vi "AlliGator Run FLI Dataset Python Function.vi"(8 "error in (no error)":errorcluster, 9 "Current Data":string, 10 "Python Function Info":T1={"Script Path"=path "", "Function Name"="", "Function Parent Menu"="", "Function Input Parameters"=[], "Function Outputs"=[], "Function Doc String"="", "Function Display Name"="", "Function Target Type"=enum."Window Menu", "Function Target Window"="", "Parent Menu Location"="", "Item Menu Tag"="", "Is preceded by Separator"=FALSE}, 11 "Data Value Reference in":refnum<data-value>) -> (0 "error out":errorcluster, 1 "Message":string, 2 "Function Output Destination":string, 3 "Data Value Reference out":refnum<data-value>)   [LabVIEW 2021, in "AlliGator Python Plugins.lvlib"]
doc: "Runs FLI Dataset python plugin function."
uses:
  AlliGator Python Plugins.lvlib
  AlliGator Internal Variables v2.ctl
  <vilib>/vision/Image Controls.llb/IMAQ Image.ctl
  AlliGator Gate Image Set.ctl
  AlliGator FLI Dataset Type.ctl
  AlliGator Data Series Type.ctl
  AlliGator Dataset Channel.ctl
  AlliGator Gate Arithmetic.ctl
  AlliGator Displayed Image.ctl
  Image/Named ROI Description.ctl
  AlliGator Decay Metadata v3.ctl
  AlliGator Decay Background Subtraction Info.ctl
  AlliGator Baseline Subtraction Method.ctl
  Graphs/XY Graph/XY Graph Plot Shift Parameters.ctl
  Graphs/XY Graph/XY Graph Plot Shift Method.ctl
  AlliGator Decay Extrapolation Parameters.ctl
  Phasor/Calibration Phasor (m, phi).ctl
  Phasor/Phasor Reference Series.ctl
  Phasor/Phasor Calibration Map v2.ctl
  Phasor/Phasor (g, s).ctl
  AlliGator Raw Phasor Plot Data v4.ctl
  Phasor/Phasor Standard Deviation Options.ctl
  AlliGator Phasor Multi-Harmonic Data.ctl
  Phasor/Phasor Harmonic Data.ctl
  AlliGator Decay Fit Options & Parameters v2.ctl
  Fits/IRF(X)PSED/Decay Fit Options v2.ctl
  Fits/Decay Convolution/Decay Model.ctl
  Fits/Residual Type.ctl
  Fits/IRF(X)PSED/Fit Weights Type.ctl
  Fits/Non-linear Fitting Method v2.ctl
  Fits/Fit Calculation Method.ctl
  Fits/Non-linear Fitting Algorithm.ctl
  AlliGator Decay Fit Parameter Constraints 2.ctl
  Fits/IRF(X)PSED/Decay Fit Parameters In List.ctl
  Fits/IRF(X)PSED/MLE Baseline Offset Type.ctl
  AlliGator Decay Preprocessing Parameters.ctl
  Fits/IRF(X)PSED/Decay Fit Parameters & Derived Quantities List.ctl
  AlliGator Python Function Information.ctl
  AlliGator Python Function Parameter Definition.ctl
  AlliGator Python Function Output Definition.ctl
  AlliGator Python Plugin Target Type.ctl
  AlliGator Variables List.ctl
  AlliGator Python Plugin FLI Dataset Data.ctl
  AlliGator Python Plugin Image Data.ctl
  AlliGator Python Plugin Plot Data.ctl
  AlliGator Python Plugin Parameter Map Data.ctl
  Image/Image Point.ctl
  <vilib>/Utility/error.llb/Error Cluster From Error Code.vi
  <vilib>/ErrorRing/Error Ring.xnode
  AlliGator Globals, Variables & Constants.lvlib
  Image/Image.lvlib
  Strings/Strings.lvlib
  Error/Error.lvlib
  Phasor/Phasor.lvlib
  AlliGator Decay Preprocessing.lvlib
  Graphs/XY Graph/XY Graph Add-Ons.lvlib
  AlliGator Phasor Graph.lvlib
  AlliGator Files.lvlib
  AlliGator Phasor Plot.lvlib
  AlliGator Source Image.lvlib
  Fits/Fits.lvlib
  AlliGator Decay Fit.lvlib
  AlliGator Decay Fit Parameter Map.lvlib
  AlliGator Internal Variables.lvlib
  AlliGator Settings.lvlib
  AlliGator Dual-Channel Datasets.lvlib
panel:
  out "session out":refnum<k35>
  out "Function Parameters String":string
  # "see the AlliGator License on the block diagram (Ctrl+E or Window:Show Block Diagram)"
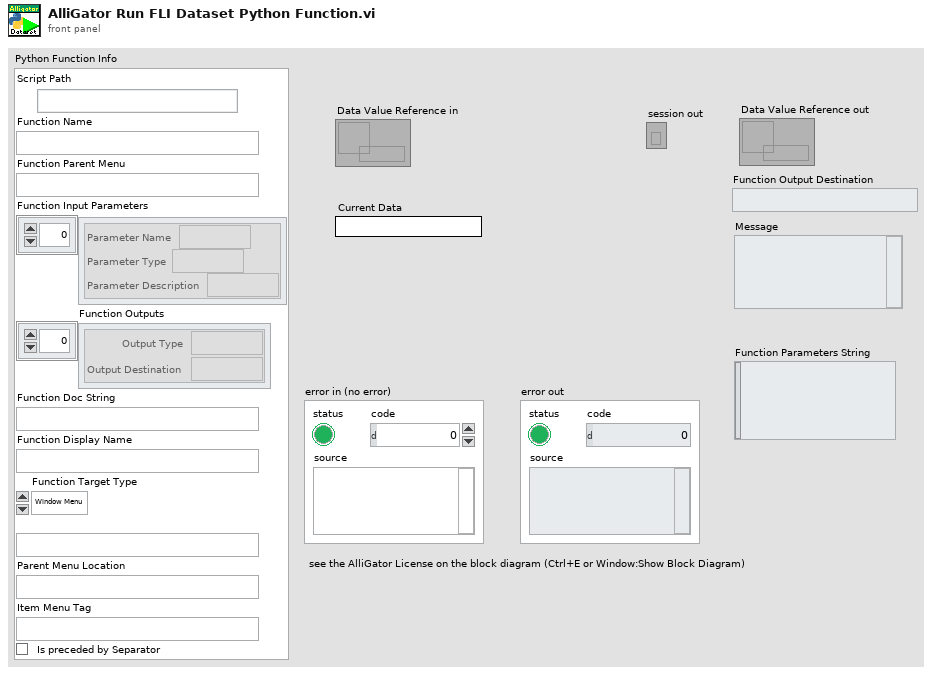
[diagram p1: front panel]
types:
  T1 = typedef "AlliGator Python Plugins.lvlib/AlliGator Python Function Information.ctl" = cluster{"Script Path":path, "Function Name":string, "Function Parent Menu":string, "Function Input Parameters":T2[], "Function Outputs":T3[], "Function Doc String":string, "Function Display Name":string, "Function Target Type":T4, "Function Target Window":string, "Parent Menu Location":string, "Item Menu Tag":string, "Is preceded by Separator":bool}
  T2 = typedef "AlliGator Python Plugins.lvlib/AlliGator Python Function Parameter Definition.ctl" = cluster{"Parameter Name":string, "Parameter Type":string, "Parameter Description":string}
  T3 = typedef "AlliGator Python Plugins.lvlib/AlliGator Python Function Output Definition.ctl" = cluster{"Output Type":string, "Output Destination":string}
  T4 = typedef "AlliGator Python Plugins.lvlib/AlliGator Python Plugin Target Type.ctl" = enum16{"Undefined", "Window Menu", "Object Menu"}
  T5 = typedef "AlliGator Python Plugins.lvlib/AlliGator Python Plugin FLI Dataset Data.ctl" = cluster{"FLI_Dataset_Name":string, "Gate_Duration":dbl, "Gate_Separation":dbl, "Gate_Number":u32, "X_Size":i32, "Y_Size":i32, "Image_Data_List":T6[], "Reference_Decay":T7, "Mask_Image":i32[][], "Parameter_Map":T8}
  T6 = typedef "AlliGator Python Plugins.lvlib/AlliGator Python Plugin Image Data.ctl" = cluster{"Image_Name":string, "Image":sgl[][]}
  T7 = typedef "AlliGator Python Plugins.lvlib/AlliGator Python Plugin Plot Data.ctl" = cluster{"Plot_Name":string, "X_Array":dbl[], "Y_Array":dbl[]}
  T8 = typedef "AlliGator Python Plugins.lvlib/AlliGator Python Plugin Parameter Map Data.ctl" = cluster{"Parameter_Names":string[], "Parameter_Flattened_Map":dbl[][], "Locations":T9[], "IRF_X":dbl[], "IRF_Y_Flattened_List":dbl[][]}
  T9 = typedef "Image.lvlib/Image Point.ctl" = cluster{"X":i32, "Y":i32}
  T10 = typedef "AlliGator Globals, Variables & Constants.lvlib/AlliGator Variables List.ctl" = enum16{"---- GUI ----", "Initialization Status", "State Indicators Refnum", "Original AlliGator Menu Items", "Current Action Loop State", "Script in progress", "Playback", "Loop Playback", "Search ROI Used", "Search ROI", "Decay Graph Max Legend Size", "Intensity Graph Max Legend Size", "Decay Statistics Graph Max Legend Size", "Phasor Graph Max Legend Size", "Phasor Ratio Graph Max Legend Size", "Lifetime Graph Max Legend Size", "---- Files ----", "Export Dataset Frames as Individual Files", "Show Batch Export Help Balloons", "Frames in Dataset", "ptu File Frame Start Indices", "Current Frame in Dataset", "Current Frame Timestamp", "------ Python Plugins ------", "Python Plugins Information", "Python Session", "Valid Python Session?", "---- Source Image ----", "Dataset Loaded", "Dataset Metadata", "Dataset Channel", "Dataset Data Description", "Background Dataset Metadata", "Background Dataset Channel", "Background Dataset Data Description", "Background File Subtraction", "Background File Path", "Background File Pile-up Correction", "Background File Pixel Well Capacity", "Background File Scaling Factor", "Source Image ROIs", "Current Source Image ROI", "Source Image ROI Event Refnum", "X_Source Image Display Range", "X_Source Image Palette Information", "Source Image Palette List", "Source Image Scale", "Current Dataset Load Settings", "Source Image:ROI Overlay Color", "---- Image Profile Window ----", "Image Profile:Overlay ROI in Source Image", "Image Profile Window Event Refnum", "Image Profile:IntensityType", "Image Profile:Intensity Average Type", "Image Profile:Intensity-weighted SDV", "Image Profile:Box Profile Type", "Image Profile Window Open", "Image Profile:Plotted Fit Parameter", "X_Type of Displayed Image", "X_Time Gate Slider", "Dataset Path", "Source Image Overlay to Erase", "Is Displayed Image Accumulated", "White Light Image Modified", "Mask Image Modified", "Macrotime Gate Separation", "------ Phasor Graph -------", "Phasor Graph:Show Line", "---- Phasor Plot ---", "Phasor Plot Parameters Changed", "FLI Dataset Modified since last Phasor Plot Calculation", "Phasor Harmonics Data", "Selected Phasor Harmonics", "Phasor Harmonic Manager Event Refnum", "Phasor Plot ROIs", "Current Phasor Plot ROI", "Phasor Plot ROI Event Refnum", "Phasor Plot Image Reference Points", "Phasor Plot Computed", "Phasor Plot Palette Information", "Phasor Plot Palette List", "Phasor Ratio Palette Information", "Phasor Ratio Palette List", "Phasor Image Scale", "Phasor Plot Image Overlay to Erase", "Phasor Plot Image Elements to Update", "Current Phasor Plot Calculation Parameters", "Current Phasor Calibration Options", "Reset Cumulated Phasor Plot", "Phasor Ratio Reference 1", "Phasor Ratio Lifetime Reference 1", "Phasor Ratio Reference 1 Frequency", "Phasor Ratio Reference 2", "Phasor Ratio Lifetime Reference 2", "Phasor Ratio Reference 2 Frequency", "---- Decay Analysis ----", "Number of Selected Decays to Fit", "LS Fit Results", "LAR Fit Results", "BS Fit Results", "Last Decay Max - Min", "Best Fit Parameters", "Best Fit Parameter Names", "Actual Size X", "Actual Size Y", "Binning X", "Binning Y", "Actual # Gates", "Dataset Number", "Gates to...", "Gates Skipped", "Gates to keep", "Gate Step", "Gate Separation", "Reversed Gates", "Pile-up Correction", "Pixel Well Capacity", "Background Subtracted", "Background Subtraction Method", "Background Definition Range", "Background File (deprecated)", "Number of Dataset Accumulated", "Array of Accumulated Dataset Paths", "Do Averaged Datasets", "Destination File Path", "Process Plot Target", "Use 1/D as Phasor Frequency", "---- Decay Fit Parameter Map -----", "Decay Fit Parameter Map Palette Information", "Decay Fit Parameter Map Palette List", "Local Decay Graph Window Event Refnum", "------- Local Decay Window ---------", "Use normalized IRF for convolution", "----- Miscellaneous ----", "Skippable Dialog Windows Status"}
  T11 = typedef "AlliGator Internal Variables.lvlib/AlliGator Internal Variables v2.ctl" = cluster{"Displayed Image":T12, "White Light Image":T12, "Mask Image":T12, "ROI Mask Image":T12, "Current Dataset Images 1":T13, "Background Dataset Images 1":T13, "Current Dataset Images 2":T13, "Background Dataset Images 2":T13, "Current Dataset Arithmetic Images":T13, "Accumulated Dataset Images 1":T13, "Accumulated Dataset Images 2":T13, "Accumulated Dataset Arithmetic Images":T13, "Phasor Plot Image":T12, "Decay Fit Parameter Map Image":T12, "Single Data Point Path":path, "White Light Image Path":path, "Mask Image Path":path, "Time-Series Folder":path, "[Time-Series Paths]":path[], "Current Dataset":i32, "Single Dataset Type":T14, "Current Folder":string, "AlliGator Data Series Type":T15, "# Datasets":i32, "Dual-Channel Dataset":bool, "Selected Channel Name":string, "Dataset Channel":T16, "Channel Arithmetic":T17, "Dual-Channel Background Dataset":bool, "Background Channel":T16, "Dual-Channel Accumulated Dataset":bool, "Start Time":dbl, "[Time-Series Timestamps]":dbl[], "[Intensity Corrections]":dbl[], "Time Series Script":bool, "Type of Displayed Image":T18, "Gate Image Slide":u16, "# Gates":i32, "ROIs":T19[], "ROI Decay":cluster{"t Array":dbl[], "I Array":dbl[]}, "Valid Decay":bool, "Decay  Metadata":T21, "Reference Decay Plot Name":string, "Reference Decay":cluster{"t Array":dbl[], "I Array":dbl[]}, "Decay Shift Plot":cluster{"Time Stamps":dbl[], "Decay Shifts":dbl[]}, "[Decays Max Values]":sgl[], "[Decays Min Values]":sgl[], "Calibration Phasor":T27, "Calibration Phasor Series":T28, "Phasor Calibration Map":T29, "Calibration Map MD5 Digest":string, "Last Raw Phasor":T30, "Last Calibrated Phasor":T30, "Last Calibrated Phasor SDV":T30, "Phasor Graph:Phasor Plot":cluster{"g Array":dbl[], "s Array":dbl[]}, "Phasor Graph:Phasor SDV Plot":cluster{"g Array":dbl[], "s Array":dbl[]}, "[Phasor Graph:Raw Phasor Plots]":T31[], "Phasor Plot locked to Ref 1":i32, "[Phasor Plot(s) locked to Ref 1]":i32[], "[Phasor Plot(s) locked to Ref 2]":i32[], "[Pixel Phasors]":T30[], "[[Sum Image]]":dbl[][], "[[CSG Phasors]]":csg[][], "[[Valid Pixel?]]":bool[][], "I/m/phi Dataset":cluster{"I/m/phi Dataset?":bool, "Base Frequency":dbl[unit], "Harmonic Orders":u8[]}, "Multi Phasor Plot Data":T33, "Decay Fit Options & Parameters":T35, "Fit Options: Decay Preprocessing Parameters":T46, "Fit Options: Reference Decay":cluster{"t Array":dbl[], "I Array":dbl[]}, "Is Full Image Parameters Map":bool, "Is Single-Pixels Parameters Map":bool, "NLSF Parameters Map X Resolution":i32, "NLSF Parameters Map Y Resolution":i32, "[Single Decay Fit Parameters]":dbl[], "Fit Model":T37, "[[Multiple Decays Fit Parameters]]":dbl[][], "[[Multiple Decays Fit Parameter SDVs]]":dbl[][], "[[IRFs]]":dbl[][], "IRF Array Time Axis":dbl[], "Decay Array Time Axis":dbl[], "[Decay Fit Parameter Names]":T47[], "[[Phasor Ratios]]":dbl[][], "[[Average Lifetimes]]":dbl[][], "Amplitude Weighted Average Lifetime":bool, "[Decay Sum]":dbl[], "[[User-defined Quantities]]":dbl[][], "User-defined Quantity":string}
  T12 = typedef "IMAQ Image.ctl" = refnum<image>
  T13 = typedef "AlliGator Files.lvlib/AlliGator Gate Image Set.ctl" = cluster{"SGL Image Max":T12, "SGL Image Sum":T12, "SGL Gate Images":T12[], "SGL Image Min":T12}
  T14 = typedef "AlliGator Files.lvlib/AlliGator FLI Dataset Type.ctl" = enum16{"HDF5 FLI Dataset", "Gate Image Folder", ".sdt FLI Dataset (Becker & Hickl)", ".ptu FLI Dataset (PicoQuant)", "SS1 FLI Dataset", "SS2 FLI Dataset", "I/m/phi Dataset", ".bin FLI Dataset (PicoQuant Binned)", ".bin FLI Dataset (Piccolo Binned)"}
  T15 = typedef "AlliGator Files.lvlib/AlliGator Data Series Type.ctl" = enum16{"Not a Supported Series", "Gate Images Folder Series", "SwissSPAD 2 Dataset Series", "B&H FLI Dataset Series", "PicoQuant PTU FLI Dataset Series", "PicoQuant BIN FLI Dataset Series", "Piccolo hist BIN FLI Dataset Series", "HDF5 FLI Dataset Series"}
  T16 = typedef "AlliGator Dual-Channel Datasets.lvlib/AlliGator Dataset Channel.ctl" = enum16{"G2", "INT"}
  T17 = typedef "AlliGator Settings.lvlib/AlliGator Gate Arithmetic.ctl" = enum16{"None", "INT-G2", "G2/INT*<INT>", "(1 - G2/INT)*<INT>"}
  T18 = typedef "AlliGator Source Image.lvlib/AlliGator Displayed Image.ctl" = enum16{"Single Gate", "Sum of All Gates", "Max of All Gates", "Min of All Gates", "-", "White Ligth Image", "Mask Image"}
  T19 = typedef "Image.lvlib/Named ROI Description.ctl" = cluster{"ROI Descriptor":T20, "ROI Name":string, "Overlay Color":u32}
  T20 = typedef "ROI Descriptor" = cluster{"Global Rectangle":i32[], "Contours":cluster{"ID":enum32{"External", "Internal"}, "Type":u32, "Coordinates":i32[]}[]}
  T21 = typedef "AlliGator Phasor Graph.lvlib/AlliGator Decay Metadata v3.ctl" = cluster{"ROI Descriptor":T20, "ROI Center":cluster{"X":i32, "Y":i32}, "Decay Background Subtraction Info":T22, "Decay Reverted":bool, "Decay Smoothened":bool, "Decay Straightened":bool, "Fitted Tau (Decay Straightening)":dbl, "Decay Shift Parameters":T24, "Decay Shifted":bool, "Decay Extrapolated":bool, "Decay Extrapolation Parameters":T26, "Decay Normalized":bool, "Fold Decay":bool, "# Folds":u32}
  T22 = typedef "AlliGator Decay Analysis.lvlib/AlliGator Decay Preprocessing.lvlib/AlliGator Decay Background Subtraction Info.ctl" = cluster{"Laser Period":dbl[unit], "Gate Duration":dbl[unit], "Baseline Subtraction Method":T23, "Background Definition Range":cluster{"Min Gate":dbl[unit], "Max Gate":dbl[unit]}, "Total Intensity w/o Bkgd Subtraction":dbl, "Bkgd-subtracted Intensity (exp)":dbl, "# Data Points":i32, "Background/Gate":dbl, "Fitted Lifetime":dbl[unit], "Bkgd-subtracted Intensity (theo)":dbl}
  T23 = typedef "AlliGator Decay Analysis.lvlib/AlliGator Decay Preprocessing.lvlib/AlliGator Baseline Subtraction Method.ctl" = enum16{"Mean", "Min", "Square Gated Single-Exponential", "File", "Constant"}
  T24 = typedef "XY Graph Add-Ons.lvlib/XY Graph Plot Shift Parameters.ctl" = cluster{"Type":T25, "Shift":dbl[unit], "Threshold":dbl, "Rotate":bool}
  T25 = typedef "XY Graph Add-Ons.lvlib/XY Graph Plot Shift Method.ctl" = enum16{"Default", "CFD", "Threshold", "Cross-Correlation"}
  T26 = typedef "AlliGator Decay Analysis.lvlib/AlliGator Decay Preprocessing.lvlib/AlliGator Decay Extrapolation Parameters.ctl" = cluster{"Additional Points":u32, "Head Fraction":dbl, "Fitted Tau":dbl, "Use Periodicity":bool, "Use Cursors":bool, "Tail Fraction":dbl}
  T27 = typedef "Phasor.lvlib/Calibration Phasor (m, phi).ctl" = cluster{"m":dbl, "phi":dbl, "Phasor Frequency":dbl[unit], "Reference Lifetime":dbl[unit]}
  T28 = typedef "Phasor.lvlib/Phasor Reference Series.ctl" = cluster{"m Array":dbl[], "phi Array":dbl[], "Phasor Frequency":dbl[unit], "Calibration Lifetime":dbl[unit]}
  T29 = typedef "AlliGator Phasor Calibration.lvlib/AlliGator Phasor Calibration Map v2.ctl" = cluster{"Phasor Frequency":dbl[unit], "Calibration Lifetime":dbl[unit], "ROI Centers":cluster{"X":i32, "Y":i32}[], "ROI Descriptors":T20[], "Map Resolution X":i32, "Map Resolution Y":i32, "z Array":cdb[]}
  T30 = typedef "Phasor.lvlib/Phasor (g, s).ctl" = cluster{"g":dbl, "s":dbl}
  T31 = typedef "AlliGator Phasor Graph.lvlib/AlliGator Raw Phasor Plot Data v4.ctl" = cluster{"Phasor Plot Name":string, "Raw Phasor Plot":T30[], "Phasor Frequency":dbl[unit], "[Decay Metadata]":T21[], "Raw Phasor Plot SDV":T30[], "Phasor SDV Options":T32, "[Calibration Phasor]":T27[]}
  T32 = typedef "Phasor.lvlib/Phasor Standard Deviation Options.ctl" = cluster{"Compute Estimated SDV":bool, "# Replicas":u32, "Use Estimated Average Phasor":bool}
  T33 = typedef "AlliGator Phasor Plot.lvlib/AlliGator Phasor Multi-Harmonic Data.ctl" = cluster{"Base Frequency":dbl[unit], "# Harmonics":u8, "Harmonic Orders":u8[], "Phasor Plot Settings Checksum":u64, "Phasor Harmonic Data Array":T34[]}
  T34 = typedef "Phasor.lvlib/Phasor Harmonic Data.ctl" = cluster{"Phasor Harmonic Name":string, "Phasor Plot Settings Checksum":u64, "Phasor Frequency":dbl[unit], "Base Frequency":dbl[unit], "Harmonic Order":u8, "Phasor Plot Parameters":string, "Phasor Array [[CSG]]":csg[][], "Dataset File Path":path}
  T35 = typedef "AlliGator Decay Fit Parameter Map.lvlib/AlliGator Decay Fit Options & Parameters v2.ctl" = cluster{"SYNC Period":dbl[unit], "Fit Options":T36, "Fit Parameter Constraints":T43[], "MLE Baseline Offset":dbl, "MLE Baseline Offset Type":T45}
  T36 = typedef "Fits.lvlib/Decay Fit Options v2.ctl" = cluster{"Show Fit Residuals":bool, "Fit Model":T37, "Residual Type":T38, "Max Decay Percentile":dbl, "Min Decay Percentile":dbl, "Show Full Decay":bool, "Weights":T39, "Fitting Method":T40, "Compute Parameter Uncertainties":bool, "Periodic Boundaries":bool, "Model Calculation":T41, "Period":dbl[unit], "Termination Criteria":cluster{"Max Iterations":i32, "Max Function Calls":i32, "Max Time":dbl[unit], "Function Tolerance":dbl, "Parameter Tolerance":dbl, "Gradient Tolerance":dbl, "Min Lambda":dbl, "Max Lambda":dbl, "Initial Tick Count":u32}, "Offset Resolution":dbl[unit], "Use Local IRF":bool, "Fitting Algorithm":T42}
  T37 = typedef "Fits.lvlib/Decay Model.ctl" = enum16{"1-Exponential", "2-Exponentials"}
  T38 = typedef "Fits.lvlib/Residual Type.ctl" = enum16{"Standard", "Normalized", "Reduced"}
  T39 = typedef "Fits.lvlib/Fit Weights Type.ctl" = enum16{"Unweighted", "1/Variance", "Best of All"}
  T40 = typedef "Fits.lvlib/Non-linear Fitting Method v2.ctl" = enum16{"Least Square", "Least Absolute Residual", "Bisquare", "MLE", "-", "Best of All"}
  T41 = typedef "Fits.lvlib/Fit Calculation Method.ctl" = enum16{"Simulation", "Convolution", "Integration"}
  T42 = typedef "Fits.lvlib/Non-linear Fitting Algorithm.ctl" = enum16{"Levenberg-Marquardt", "Trust-Region Dogleg"}
  T43 = typedef "AlliGator Decay Analysis.lvlib/AlliGator Decay Fit.lvlib/AlliGator Decay Fit Parameter Constraints 2.ctl" = cluster{"Fit Parameter":T44, "Min Value":dbl, "Max Value":dbl, "Global":bool, "Used":bool}
  T44 = typedef "Fits.lvlib/Decay Fit Parameters In List.ctl" = enum16{"Offset", "Baseline", "A_1", "tau_1", "A_2", "tau_2"}
  T45 = typedef "AlliGator Settings.lvlib/MLE Baseline Offset Type.ctl" = enum32{"Absolute", "Percentage"}
  T46 = typedef "AlliGator Decay Analysis.lvlib/AlliGator Decay Preprocessing.lvlib/AlliGator Decay Preprocessing Parameters.ctl" = cluster{"Background Subtraction":bool, "Straighten Decay":bool, "Reverse Gates":bool, "1-Normalized Decay":bool, "Smoothen Decay":bool, "Smoothing Parameter":dbl, "Shift Decay":bool, "Decay Shift Parameters":T24, "Extrapolate Decay":bool, "Additional Points":u32, "Head Fraction":dbl, "Pixel-Normalize Decay":bool, "Use Periodicity":bool, "Use Cursors":bool, "Tail Fraction":dbl, "Use Decay Pre-Processing":bool, "Fold Decay":bool, "# Folds":u32, "[0-1]-Normalized Decay":bool}
  T47 = typedef "Fits.lvlib/Decay Fit Parameters & Derived Quantities List.ctl" = enum16{"Offset", "Baseline", "A_1", "tau_1", "A_2", "tau_2", "<tau>_a", "f1_a", "f2_a", "<tau>_i", "f1_i", "f2_i", "-", "R^2", "Chi^2"}
  T48 = typedef "Image Type" = u32
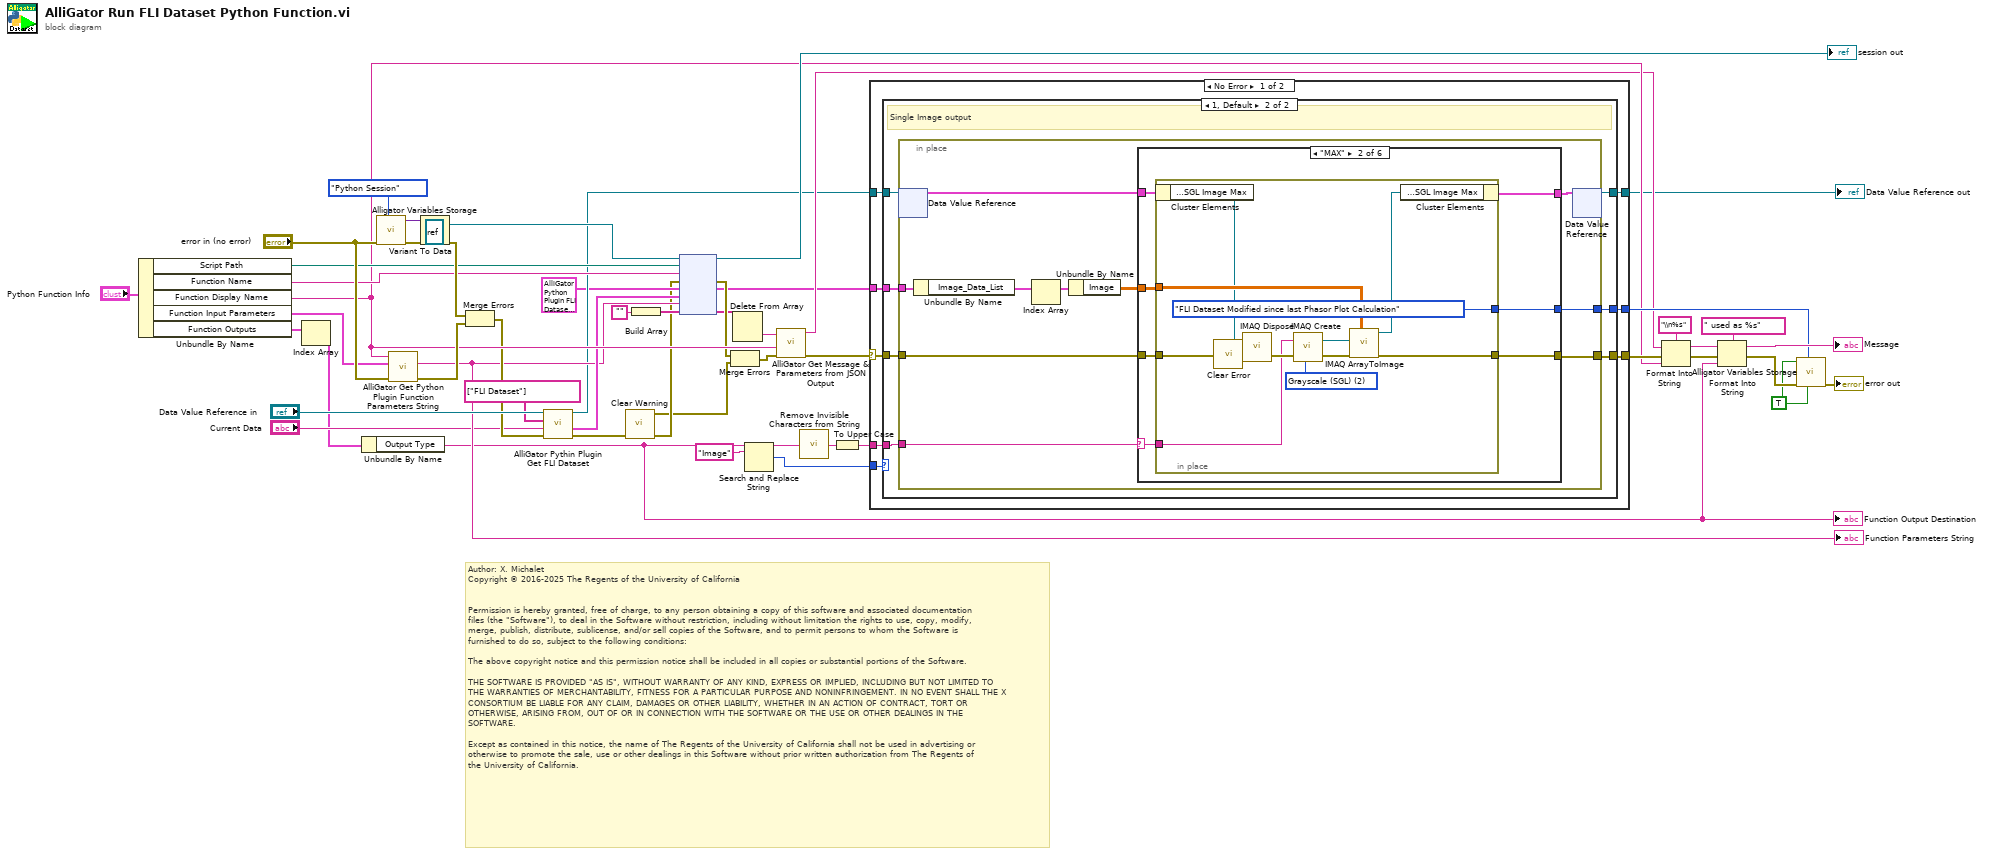
[diagram p0: block diagram]
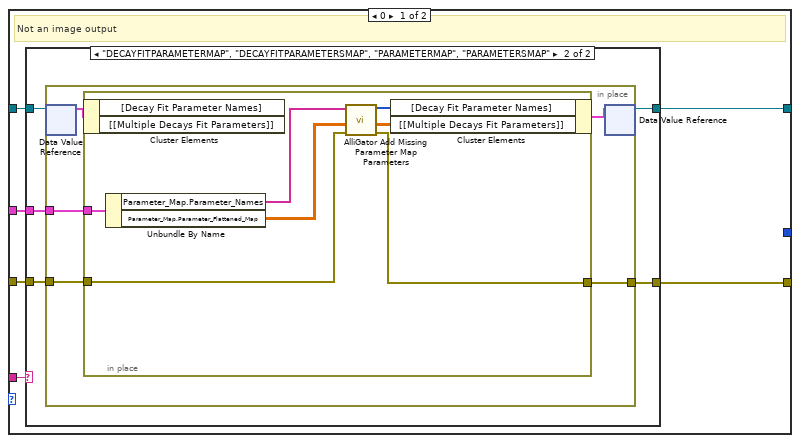
[diagram p2: hidden frame]
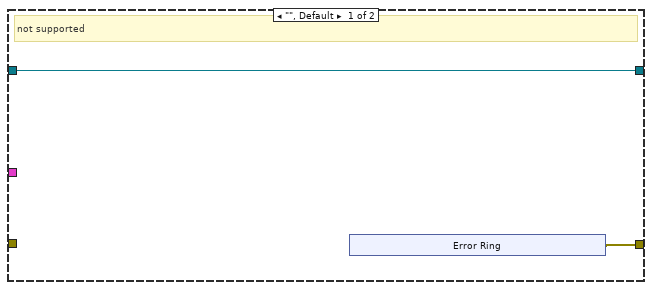
[diagram p3: hidden frame]
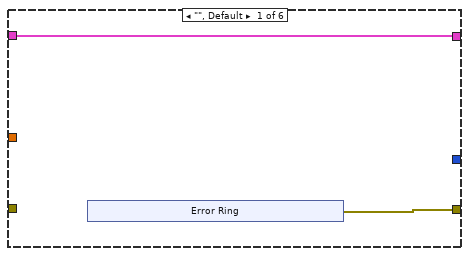
[diagram p4: hidden frame]
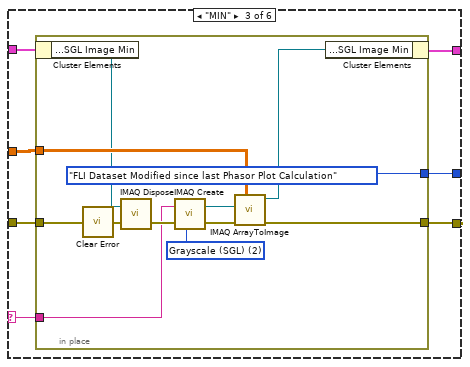
[diagram p5: hidden frame]
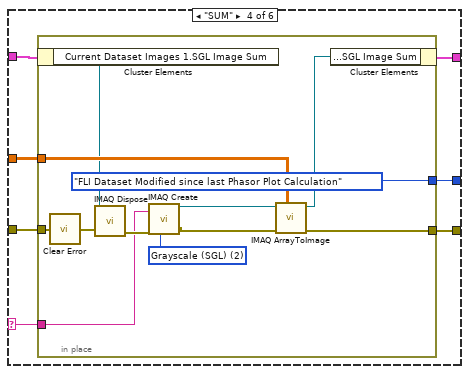
[diagram p6: hidden frame]
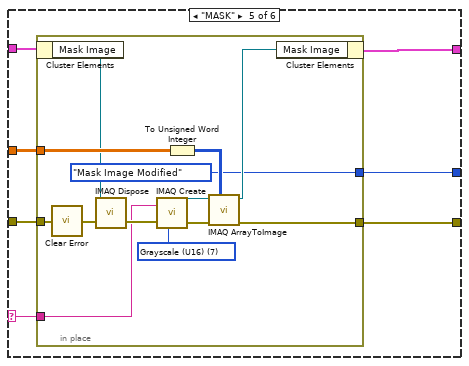
[diagram p7: hidden frame]
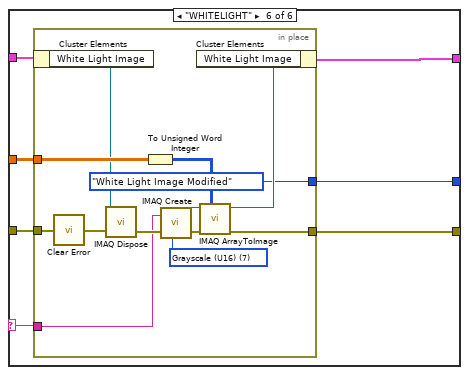
[diagram p8: hidden frame]
diagram:
  w35 = TRUE ("Get(F)/Set")
  # "Author: X. Michalet\nCopyright © 2016-2025 The Regents of the University of California\n \n\nPermission is hereby granted, free of charge, to any person obtaining a copy of this software and associated documentation files (the \"Software\"), to deal in the Software without restriction, including without limitation the rights to use, copy, modify, merge, publish, distribute, sublicense, and/or sell copies of the Software, and to permit persons to whom the Software is furnished to do so, subject to the following conditions:\n\nThe above copyright notice and this permission notice shall be included in all copies or substantial portions of the Software.\n\nTHE SOFTWARE IS PROVIDED \"AS IS\", WITHOUT WARRANTY OF ANY KIND, EXPRESS OR IMPLIED, INCLUDING BUT NOT LIMITED TO THE WARRANTIES OF MERCHANTABILITY, FITNESS FOR A PARTICULAR PURPOSE AND NONINFRINGEMENT. IN NO EVENT SHALL THE X CONSORTIUM BE LIABLE FOR ANY CLAIM, DAMAGES OR OTHER LIABILITY, WHETHER IN AN ACTION OF CONTRACT, TORT OR OTHERWISE, ARISING FROM, OUT OF OR IN CONNECTION WITH THE SOFTWARE OR THE USE OR OTHER DEALINGS IN THE SOFTWARE.\n\nExcept as contained in this notice, the name of The Regents of the University of California shall not be used in advertising or otherwise to promote the sale, use or other dealings in this Software without prior written authorization from The Regents of the University of California."
  n1 = Unbundle By Name("Python Function Info") -> ("Script Path"=w33:path, "Function Name"=w32:string, "Function Display Name"=w30:string, "Function Input Parameters"=w31:T2[], "Function Outputs"=w10:T3[])
  n2 = Index Array(array=w10) -> (element=w9:T3)  [unwired: 1 in]
  n3 = Unbundle By Name(w9) -> ("Output Type"=w8:string)
  "Function Output Destination" <- w8
  n4 = call "Alligator Variables Storage.vi"("AlliGator Variable"=AlliGator_Variables_List."Python Session" ("Alligator Variable"), "Error In"="error in (no error)") -> ("Error Out"=w49:errorcluster, "Data out"=w47:variant)  [unwired: 7 in, 1 out]
  n5 = call "AlliGator Get Python Plugin Function Parameters String.vi"("error in (no error)"="error in (no error)", "Function Parameters"=w31, "Function Display Name"=w30) -> ("error out"=w51:errorcluster, "Function Parameters JSON String"=w21:string)  [unwired: 6 in, 1 out]
  "Function Parameters String" <- w21
  n6 = Variant To Data(error in=w49, type=refnum<k35> refnum ("session in"), Variant=w47) -> (data=w45:refnum<k35>, error out=w48:errorcluster)
  n7 = Merge Errors(w48, w51) -> (w23:errorcluster)
  n8 = call "AlliGator Pythin Plugin Get FLI Dataset.vi"("error in (no error)"=w23, "Current Data"="Current Data", "AlliGator Parameter Names Not Found"=string[] ["FLI Dataset"], "Data Value Reference in"="Data Value Reference in") -> ("error out"=w4:errorcluster, "FLI_Dataset_Data"=w22:T5, "Data Value Reference out"=w20:refnum<data-value>)  [unwired: 4 in, 1 out]
  n9 = call "Clear Warning.vi"("error in (no error)"=w4) -> ("cleared warning or error dup"=w3:errorcluster, "error in (dup)"=w1:errorcluster)  [unwired: 9 in]
  n10 = Build Array("") -> (w11:string[])
  n11 = node(w45, w33, w32, w3, T5 {"FLI_Dataset_Name"="", "Gate_Duration"=0.0, "Gate_Separation"=0.0, "Gate_Number"=0, "X_Size"=0, "Y_Size"=0, "Image_Data_List"=[], "Reference_Decay"={"Plot_Name"="", "X_Array"=[], "Y_Array"=[]}, "Mask_Image"=[], "Parameter_Map"={"Parameter_Names"=[], "Parameter_Flattened_Map"=[], "Locations"=[], "IRF_X"=[], "IRF_Y_Flattened_List"=[]}} ("FLI_Dataet_Data"), w22, w21, w11) -> (→"session out":refnum<k35>, w27:errorcluster, w15:T5, w25:string[])  [unwired: 2 in, 2 out]
  n12 = Merge Errors(w27, w1) -> (w2:errorcluster)
  n13 = Delete From Array(array=w25) -> (deleted portion=w28:string)  [unwired: 2 in, 1 out]
  n14 = Search and Replace String(input string=w8, search string="Image") -> (result string=w7:string, number of replacements=w13:i32)  [unwired: 6 in, 2 out]
  n15 = call "AlliGator Get Message & Parameters from JSON Output.vi"("error in (no error)"=w2, "Function Display Name"=w30, "<JSON>"=w28) -> ("error out"=w26:errorcluster, "Notebook Message"=w29:string)  [unwired: 7 in]
  n16 = call "Remove Invisible Characters from String.vi"("String"=w7) -> ("result string"=w6:string)  [unwired: 3 in]
  n17 = To Upper Case(1:w6) -> (0:w5:string)
  n18 = case shown="No Error" w26 {
    selector: w26 -> [w59 w212]
    tunnel: [w61 w212] -> w53
    tunnel: [w60 _] -> w36
    tunnel: w20 -> [w58 w211]
    tunnel: [w57 w211] -> w19
    tunnel: w15 -> [w56 _]
    tunnel: w13 -> [w55 _]
    tunnel: w5 -> [w54 _]
    frame No Error {
      n19 = case shown="1, Default" w55 {
        tunnel: [w65 w97] -> w61
        tunnel: [_ w96] -> w60
        tunnel: w59 -> [w64 w95]
        tunnel: w58 -> [w67 w94]
        tunnel: [w66 w93] -> w57
        tunnel: w56 -> [w63 w92]
        tunnel: w54 -> [w62 w91]
        frame 0 {
          # "Not an image output"
          n20 = case shown="\"DECAYFITPARAMETERMAP\", \"DECAYFITPARAMETERSMAP\", \"PARAMETERMAP\", \"PARAMETERSMAP\"" w62 {
            tunnel: w67 -> [w69 w78]
            tunnel: [w69 w77] -> w66
            tunnel: [w68 w74] -> w65
            tunnel: w64 -> [_ w75]
            tunnel: w63 -> [_ w76]
            frame "", Default {
              # "not supported"
              n21 = xnode "Error Ring"() -> ("error out"=w68:errorcluster)
            }
            frame "DECAYFITPARAMETERMAP", "DECAYFITPARAMETERSMAP", "PARAMETERMAP", "PARAMETERSMAP" {
              n22 = in-place {
                in-place-border: w76 -> [w82]
                in-place-border: w75 -> [w80]
                in-place-border: [w79] -> w74
                n23 = in-place-dvr #1(w78) -> (w83:T11)  [unwired: 1 out]
                n24 = in-place {
                  in-place-border: w82 -> [w90]
                  in-place-border: w80 -> [w85]
                  in-place-border: [w84] -> w79
                  n25 = in-place-cluster #2(w83) -> ()  [unwired: 2 out]
                  n26 = Unbundle By Name(w90) -> ("Parameter_Map.Parameter_Names"=w86:string[], "Parameter_Map.Parameter_Flattened_Map"=w89:dbl[][])
                  n27 = call "AlliGator Add Missing Parameter Map Parameters.vi"("Error In"=w85, "Parameter_Flattened_Map in"=w89, "Parameter Names"=w86) -> ("Error Out"=w84:errorcluster, "Parameter_Flattened_Map out"=w88:dbl[][], "[Decay Fit Parameter Name] out"=w87:T47[])  [unwired: 6 in]
                  n28 = in-place-cluster #2("[Decay Fit Parameter Names]"=w87, "[[Multiple Decays Fit Parameters]]"=w88) -> (w81:T11)
                }
                n29 = in-place-dvr #1(w81) -> (w77:refnum<data-value>)  [unwired: 1 out]
              }
            }
          }
        }
        frame 1, Default {
          # "Single Image output"
          n30 = in-place {
            in-place-border: [w107] -> w97
            in-place-border: [w106] -> w96
            in-place-border: w91 -> [w98]
            in-place-border: w95 -> [w105]
            in-place-border: w92 -> [w102]
            n31 = in-place-dvr #3(w94) -> (w104:T11)  [unwired: 1 out]
            n32 = Unbundle By Name(w102) -> ("Image_Data_List"=w101:T6[])
            n33 = Index Array(array=w101) -> (element=w100:T6)  [unwired: 1 in]
            n34 = Unbundle By Name(w100) -> ("Image"=w99:sgl[][])
            n35 = case shown="\"MAX\"" w98 {
              selector: w98 -> [_ w116 w135 w155 w172 w193]
              tunnel: w104 -> [w109 w120 w139 w158 w177 w197]
              tunnel: w99 -> [_ w119 w138 w153 w176 w196]
              tunnel: [w109 w118 w137 w157 w175 w195] -> w103
              tunnel: [w108 w117 w136 w156 w174 w194] -> w107
              tunnel: w105 -> [_ w115 w134 w154 w173 w192]
              tunnel: [_ w114 w133 w152 w171 w191] -> w106
              frame "", Default {
                n36 = xnode "Error Ring"() -> ("error out"=w108:errorcluster)
              }
              frame "MAX" {
                n37 = in-place {
                  in-place-border: w119 -> [w131]
                  in-place-border: w115 -> [w128]
                  in-place-border: [w130] -> w117
                  in-place-border: w116 -> [w123]
                  in-place-border: [AlliGator_Variables_List."FLI Dataset Modified since last Phasor Plot Calculation" ("Alligator Variable")] -> w114
                  w124 = T48 2 items=["Grayscale (U8)", "Grayscale (I16)", "Grayscale (SGL)", "Complex (CSG)", "RGB (U32)", "HSL (U32)", "RGB (U64)", "Grayscale (U16)"] ("Image Type")
                  n38 = in-place-cluster #4(w120) -> ("Current Dataset Images 1.SGL Image Max"=w129:T12)
                  n39 = call "Clear Error.vi"("Error In"=w128) -> ("no Error Out"=w121:errorcluster)  [unwired: 8 in]
                  n40 = call "IMAQ Dispose"("Image"=w129, "error in (no error)"=w121) -> ("error out"=w127:errorcluster)  [unwired: 4 in]
                  n41 = call "IMAQ Create"("Image Name"=w123, "Image Type"=w124, "error in (no error)"=w127) -> ("New Image"=w125:T12, "error out"=w126:errorcluster)  [unwired: 2 in]
                  n42 = call "IMAQ ArrayToImage"("Image Pixels (Float)"=w131, "error in (no error)"=w126, "Image"=w125) -> ("error out"=w130:errorcluster, "Image Out"=w132:T12)  [unwired: 7 in]
                  n43 = in-place-cluster #4("Current Dataset Images 1.SGL Image Max"=w132) -> (w118:T11)
                }
              }
              frame "MIN" {
                n44 = in-place {
                  in-place-border: w138 -> [w150]
                  in-place-border: w134 -> [w147]
                  in-place-border: [w149] -> w136
                  in-place-border: w135 -> [w142]
                  in-place-border: [AlliGator_Variables_List."FLI Dataset Modified since last Phasor Plot Calculation" ("Alligator Variable")] -> w133
                  w143 = T48 2 items=["Grayscale (U8)", "Grayscale (I16)", "Grayscale (SGL)", "Complex (CSG)", "RGB (U32)", "HSL (U32)", "RGB (U64)", "Grayscale (U16)"] ("Image Type")
                  n45 = in-place-cluster #5(w139) -> ("Current Dataset Images 1.SGL Image Min"=w148:T12)
                  n46 = call "Clear Error.vi"("Error In"=w147) -> ("no Error Out"=w140:errorcluster)  [unwired: 8 in]
                  n47 = call "IMAQ Dispose"("Image"=w148, "error in (no error)"=w140) -> ("error out"=w146:errorcluster)  [unwired: 4 in]
                  n48 = call "IMAQ Create"("Image Name"=w142, "Image Type"=w143, "error in (no error)"=w146) -> ("New Image"=w144:T12, "error out"=w145:errorcluster)  [unwired: 2 in]
                  n49 = call "IMAQ ArrayToImage"("Image Pixels (Float)"=w150, "error in (no error)"=w145, "Image"=w144) -> ("error out"=w149:errorcluster, "Image Out"=w151:T12)  [unwired: 7 in]
                  n50 = in-place-cluster #5("Current Dataset Images 1.SGL Image Min"=w151) -> (w137:T11)
                }
              }
              frame "SUM" {
                n51 = in-place {
                  in-place-border: w153 -> [w169]
                  in-place-border: [w168] -> w156
                  in-place-border: w155 -> [w162]
                  in-place-border: w154 -> [w161]
                  in-place-border: [AlliGator_Variables_List."FLI Dataset Modified since last Phasor Plot Calculation" ("Alligator Variable")] -> w152
                  w166 = T48 2 items=["Grayscale (U8)", "Grayscale (I16)", "Grayscale (SGL)", "Complex (CSG)", "RGB (U32)", "HSL (U32)", "RGB (U64)", "Grayscale (U16)"] ("Image Type")
                  n52 = in-place-cluster #6(w158) -> ("Current Dataset Images 1.SGL Image Sum"=w165:T12)
                  n53 = call "Clear Error.vi"("Error In"=w161) -> ("no Error Out"=w159:errorcluster)  [unwired: 8 in]
                  n54 = call "IMAQ Dispose"("Image"=w165, "error in (no error)"=w159) -> ("error out"=w167:errorcluster)  [unwired: 4 in]
                  n55 = call "IMAQ Create"("Image Name"=w162, "Image Type"=w166, "error in (no error)"=w167) -> ("New Image"=w163:T12, "error out"=w164:errorcluster)  [unwired: 2 in]
                  n56 = call "IMAQ ArrayToImage"("Image Pixels (Float)"=w169, "error in (no error)"=w164, "Image"=w163) -> ("error out"=w168:errorcluster, "Image Out"=w170:T12)  [unwired: 7 in]
                  n57 = in-place-cluster #6("Current Dataset Images 1.SGL Image Sum"=w170) -> (w157:T11)
                }
              }
              frame "MASK" {
                n58 = in-place {
                  in-place-border: w176 -> [w190]
                  in-place-border: [w188] -> w174
                  in-place-border: w173 -> [w180]
                  in-place-border: w172 -> [w184]
                  in-place-border: [AlliGator_Variables_List."Mask Image Modified" ("Alligator Variable")] -> w171
                  w181 = T48 7 items=["Grayscale (U8)", "Grayscale (I16)", "Grayscale (SGL)", "Complex (CSG)", "RGB (U32)", "HSL (U32)", "RGB (U64)", "Grayscale (U16)"] ("Image Type")
                  n59 = in-place-cluster #7(w177) -> ("Mask Image"=w183:T12)
                  n60 = call "Clear Error.vi"("Error In"=w180) -> ("no Error Out"=w178:errorcluster)  [unwired: 8 in]
                  n61 = call "IMAQ Dispose"("Image"=w183, "error in (no error)"=w178) -> ("error out"=w186:errorcluster)  [unwired: 4 in]
                  n62 = call "IMAQ Create"("Image Name"=w184, "Image Type"=w181, "error in (no error)"=w186) -> ("New Image"=w182:T12, "error out"=w185:errorcluster)  [unwired: 2 in]
                  n63 = To Unsigned Word Integer(number=w190) -> (unsigned 16bit integer=w187:u16[][])
                  n64 = call "IMAQ ArrayToImage"("Image Pixels (U16)"=w187, "error in (no error)"=w185, "Image"=w182) -> ("error out"=w188:errorcluster, "Image Out"=w189:T12)  [unwired: 7 in]
                  n65 = in-place-cluster #7("Mask Image"=w189) -> (w175:T11)
                }
              }
              frame "WHITELIGHT" {
                n66 = in-place {
                  in-place-border: w196 -> [w209]
                  in-place-border: [w208] -> w194
                  in-place-border: w193 -> [w205]
                  in-place-border: w192 -> [w201]
                  in-place-border: [AlliGator_Variables_List."White Light Image Modified" ("Alligator Variable")] -> w191
                  w204 = T48 7 items=["Grayscale (U8)", "Grayscale (I16)", "Grayscale (SGL)", "Complex (CSG)", "RGB (U32)", "HSL (U32)", "RGB (U64)", "Grayscale (U16)"] ("Image Type")
                  n67 = in-place-cluster #8(w197) -> ("White Light Image"=w203:T12)
                  n68 = call "Clear Error.vi"("Error In"=w201) -> ("no Error Out"=w198:errorcluster)  [unwired: 8 in]
                  n69 = call "IMAQ Dispose"("Image"=w203, "error in (no error)"=w198) -> ("error out"=w207:errorcluster)  [unwired: 4 in]
                  n70 = To Unsigned Word Integer(number=w209) -> (unsigned 16bit integer=w200:u16[][])
                  n71 = call "IMAQ Create"("Image Name"=w205, "Image Type"=w204, "error in (no error)"=w207) -> ("New Image"=w202:T12, "error out"=w206:errorcluster)  [unwired: 2 in]
                  n72 = call "IMAQ ArrayToImage"("Image Pixels (U16)"=w200, "error in (no error)"=w206, "Image"=w202) -> ("error out"=w208:errorcluster, "Image Out"=w210:T12)  [unwired: 7 in]
                  n73 = in-place-cluster #8("White Light Image"=w210) -> (w195:T11)
                }
              }
            }
            n74 = in-place-dvr #3(w103) -> (w93:refnum<data-value>)  [unwired: 1 out]
          }
        }
      }
    }
    frame Error {
    }
  }
  "Data Value Reference out" <- w19
  n75 = Format Into String(format string="\\n%s", initial string=w29, error in=w53, w30) -> (resulting string=w40:string, error out=w39:errorcluster)
  n76 = Format Into String(format string=" used as %s", initial string=w40, error in=w39, w8) -> (resulting string=→"Message":string, error out=w38:errorcluster)
  n77 = call "Alligator Variables Storage.vi"("Get(F)/Set"=w35, "AlliGator Variable"=w36, "Error In"=w38, "Data in"=w35) -> ("Error Out"=→"error out":errorcluster)  [unwired: 5 in, 2 out]
